vi "Shooter Wheel Control.vi"(11 "Shooter Wheel DevRef Out":T1) -> ()   [LabVIEW 2015, in "Shooter Wheel.lvlib"]
uses:
  <userlib>/836 Library/Motion Control/Shooter Wheel/Shooter Wheel.lvlib
  <userlib>/836 Library/Motion Control/Shooter Wheel/ShooterControl.ctl
  <userlib>/836 Library/Motion Control/Shooter Wheel/ShooterConfig.ctl
  <userlib>/836 Library/Motion Control/Shooter Wheel/ShooterData.ctl
  <vilib>/Rock Robotics/WPI/MotorControl/WPI_MotorControlDeviceRef.ctl
  <vilib>/Rock Robotics/WPI/MotorControl/WPI_MotorControlType.ctl
  <vilib>/Rock Robotics/SystemInterfaces/DIO/FPGA_DIOPWMChannel.ctl
  <vilib>/Rock Robotics/WPI/PWM/WPI_PWMDeadband.ctl
  <vilib>/Rock Robotics/WPI/CAN/Jaguar/SubVIs/WPI_CANJaguar_ControlMode.ctl
  <vilib>/Rock Robotics/WPI/CAN/TalonSRX/WPI_CANTalonSRX_APIControlMode.ctl
  <vilib>/Rock Robotics/WPI/PWM/WPI_PWMTransform_ConPane.ctl
  <vilib>/Rock Robotics/WPI/Counter/WPI_CounterDevRef.ctl
  <vilib>/Rock Robotics/SystemInterfaces/Counter/FPGA_CounterCtrSystemIndex.ctl
  <vilib>/Platform/TimedLoop/XDataNode/timing_clust.ctl
  <vilib>/Platform/TimedLoop/XDataNode/nitl_modes.ctl
  <vilib>/Platform/TimedLoop/XDataNode/wakeup.ctl
  <vilib>/Platform/TimedLoop/XDataNode/XDataNode.xnode
  <vilib>/Platform/TimedLoop/XDataNode/XDNodeRunTimeDep.lvlib
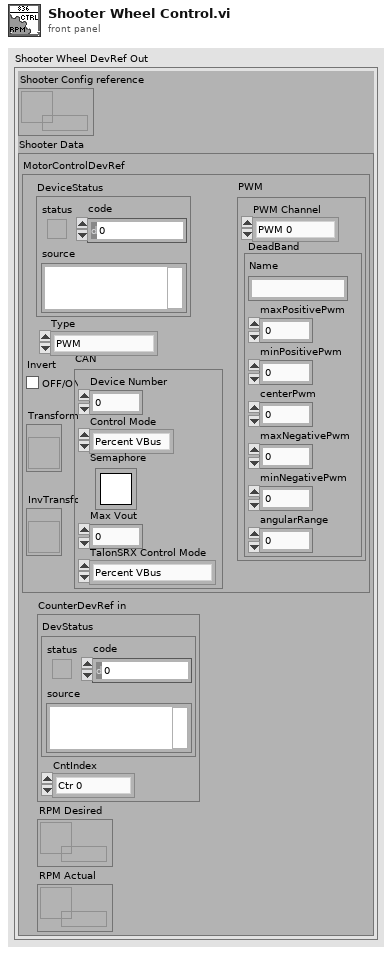
[diagram p1: front panel]
types:
  T1 = typedef "Shooter Wheel.lvlib/ShooterControl.ctl" = cluster{"Shooter Config reference":refnum<data-value>, "Shooter Data":T2}
  T2 = typedef "Shooter Wheel.lvlib/ShooterData.ctl" = cluster{"MotorControlDevRef":T3, "CounterDevRef in":T11, "RPM Desired":refnum<k33>, "RPM Actual":refnum<k33>}
  T3 = typedef "WPI_MotorControlDeviceRef.ctl" = cluster{"DeviceStatus":errorcluster, "Type":T4, "PWM":cluster{"PWM Channel":T5, "DeadBand":T6}, "CAN":cluster{"Device Number":u8, "Control Mode":T7, "Semaphore":T8, "Max Vout":dbl, "TalonSRX Control Mode":T9}, "Invert":bool, "TransformRef":T10, "InvTransformRef":T10}
  T4 = typedef "WPI_MotorControlType.ctl" = enum16{"PWM", "CAN", "CANTalonSRX"}
  T5 = typedef "FPGA_DIOPWMChannel.ctl" = enum8{"PWM 0", "PWM 1", "PWM 2", "PWM 3", "PWM 4", "PWM 5", "PWM 6", "PWM 7", "PWM 8", "PWM 9", "PWM MXP 0", "PWM MXP 1", "PWM MXP 2", "PWM MXP 3", "PWM MXP 4", "PWM MXP 5", "PWM MXP 6", "PWM MXP 7", "PWM MXP 8", "PWM MXP 9", "Invalid"}
  T6 = typedef "WPI_PWMDeadband.ctl" = cluster{"Name":string, "maxPositivePwm":i32, "minPositivePwm":i32, "centerPwm":i32, "maxNegativePwm":i32, "minNegativePwm":i32, "angularRange":u16}
  T7 = typedef "WPI_CANJaguar_ControlMode.ctl" = enum8{"Percent VBus", "Current", "Speed", "Position", "Voltage"}
  T8 = typedef "Semaphore RefNum" = refnum<k1>
  T9 = typedef "WPI_CANTalonSRX_APIControlMode.ctl" = enum8{"Percent VBus", "Speed", "Position", "Slave", "Unchanged / Invalid"}
  T10 = typedef "WPI_PWMTransform_ConPane.ctl" = refnum<vi>
  T11 = typedef "WPI_CounterDevRef.ctl" = cluster{"DevStatus":errorcluster, "CntIndex":T12}
  T12 = typedef "FPGA_CounterCtrSystemIndex.ctl" = enum8{"Ctr 0", "Ctr 1", "Ctr 2", "Ctr 3", "Ctr 4", "Ctr 5", "Ctr 6", "Ctr 7", "Invalid"}
  T13 = typedef "XDNodeRunTimeDep.lvlib/timing_clust.ctl" = cluster{"Expected End [f-1]":u64, "Actual End [f-1]":u64, "Finished Late? [f-1]":bool, "Expected End [i-1]":u64, "Actual End [i-1]":u64, "Finished Late? [i-1]":bool, "Expected Start [i]":u64, "Actual Start [i]":u64, "Expected Start [f]":u64, "Actual Start [f]":u64, "Source Name":string, "Structure Name":string, "Period":i64, "Deadline":i64, "Offset":i64, "Start":i64, "Priority":i32, "Timeout":i32, "Mode":T14, "Wakeup Reason":T15, "Error":errorcluster, "Source Type":string, "Secondary Source Type":string, "Global End Time":u64, "Global Start Time":u64, "Frame Duration":u64, "Iteration Duration":u64, "Assigned CPU":i32, "I/O Scan Engine Mode":u32}
  T14 = typedef "XDNodeRunTimeDep.lvlib/nitl_modes.ctl" = enum32{"No Change", "Process missed periods, maintain original phase", "Discard missed periods, maintain original phase", "Process missed periods, ignore original phase", "Discard missed periods, ignore original phase"}
  T15 = typedef "XDNodeRunTimeDep.lvlib/wakeup.ctl" = enum32{"Normal", "Aborted", "Asynchronous wakeup", "Timing source error", "Timed loop error", "Timeout"}
  T16 = typedef "Shooter Wheel.lvlib/ShooterConfig.ctl" = cluster{"Period (ms)":i64, "TBH Gain":dbl, "Priority":i32}
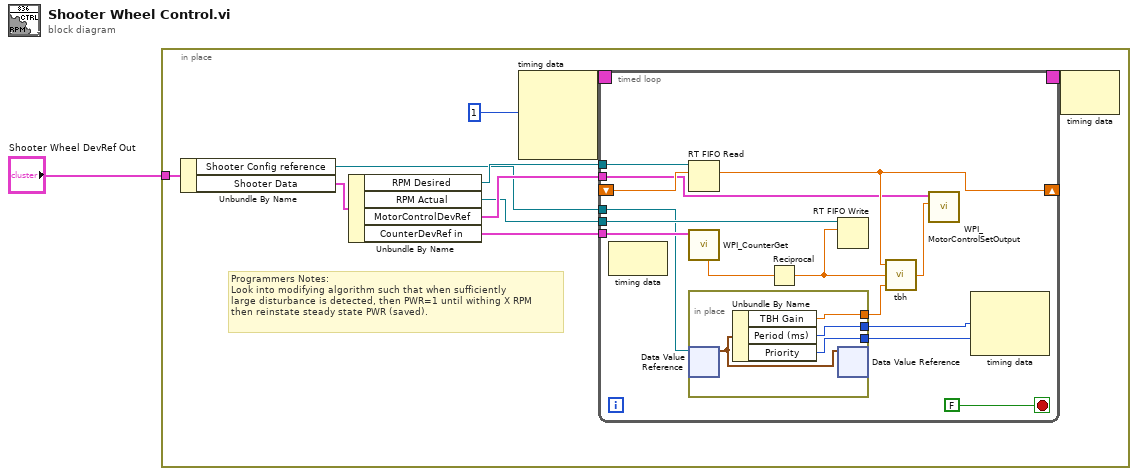
[diagram p0: block diagram]
diagram:
  n1 = in-place {
    in-place-border: "Shooter Wheel DevRef Out" -> [w2]
    # "Programmers Notes:\nLook into modifying algorithm such that when sufficiently\nlarge disturbance is detected, then PWR=1 until withing X RPM\nthen reinstate steady state PWR (saved)."
    n2 = Unbundle By Name(w2) -> ("Shooter Config reference"=w3:refnum<data-value>, "Shooter Data"=w4:T2)
    n3 = Unbundle By Name(w4) -> ("RPM Desired"=w6:refnum<k33>, "RPM Actual"=w7:refnum<k33>, "MotorControlDevRef"=w9:T3, "CounterDevRef in"=w5:T11)
    n4 = node-c288(i64 1 ("Period")) -> (w11:T13)  [unwired: 3 in]
    n5 = timed-loop {
      timing: w11 -> [_]
      timing-out: [_] -> w10
      tunnel: w6 -> [w24]
      tunnel: w7 -> [w23]
      shift-right: [w21] -> _
      shift-left: _ -> [w22]
      tunnel: w9 -> [w19]
      tunnel: w5 -> [w18]
      tunnel: w3 -> [w15]
      stop <- FALSE stop-if-true
      n6 = node-c288() -> ()  [unwired: 1 in, 1 out]
      n7 = RT FIFO Read(0:w24, 1:w22) -> (9:w21:dbl)  [unwired: 2 in, 4 out]
      n8 = call <vilib>:"WPI_CounterGet.vi"("CounterDevRef in"=w18) -> ("Period (sec)"=w17:dbl)  [unwired: 5 in, 5 out]
      n9 = in-place {
        in-place-border: [w29] -> w14
        in-place-border: [w28] -> w13
        in-place-border: [w27] -> w12
        n10 = in-place-dvr #1(w15) -> (w26:T16)  [unwired: 1 out]
        n11 = Unbundle By Name(w26) -> ("TBH Gain"=w29:dbl, "Period (ms)"=w28:i64, "Priority"=w27:i32)
        n12 = in-place-dvr #1(w26) -> ()  [unwired: 2 out]
      }
      n13 = Reciprocal(x=w17) -> (1/x=w16:dbl)
      n14 = RT FIFO Write(0:w23, 1:w16) -> ()  [unwired: 3 in, 4 out]
      n15 = call <userlib>:"tbh.vi"("Gain"=w14, "Act"=w16, "Cmd"=w21) -> ("Out"=w20:dbl)
      n16 = call <vilib>:"WPI_MotorControlSetOutput.vi"("Output"=w20, "MotorControlDevRef"=w19) -> ()  [unwired: 7 in, 3 out]
      n17 = node-c288(w13, w12) -> ()  [unwired: 1 in, 1 out]
    }
    n18 = node-c288(w10) -> ()  [unwired: 1 out]
  }
